vi "GetSettings.vi"(8 "error in (no error)":errorcluster, 10 "SettingsToRetrieve":variant, 11 "PacificPowerSource in":refnum<class "PacificPowerSource.lvclass">) -> (0 "error out":errorcluster, 1 "DeviceConfig&Meas":variant, 2 "RetrievedSettings":variant, 3 "PacificPowerSource Out":refnum<class "PacificPowerSource.lvclass">)   [LabVIEW 2018, in "AcPwrPlugins.lvlib" / "PacificPowerSource.lvclass"]
doc: "This VI retrieves a boolean status to see if the instrument can conduct measurements while the device is changing modes or turning off and on."
uses:
  PacificPowerSource.lvclass
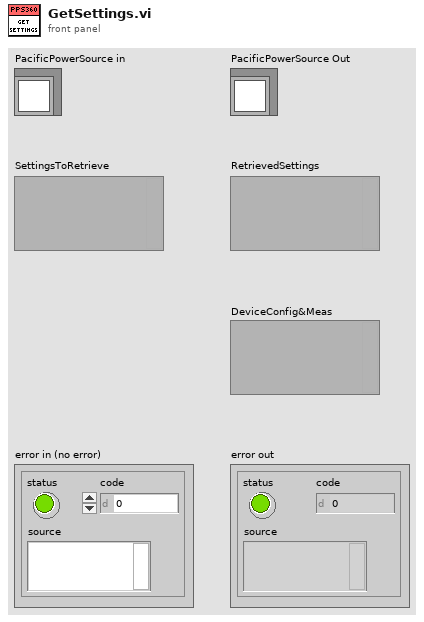
[diagram p1: front panel]
types:
  T1 = typedef "AcPwrPlugins.lvlib/PacificPowerSource.lvclass/Device(s)Settings.ctl" = cluster{"MeasName":string, "Modules":cluster{"Handle":string, "Connected":bool, "Clear Device (F)":bool, "btnIdQuery":bool, "btnReset":bool, "Program #":cluster{"Phase B (Degrees)":i32, "Waveform A (1: Sine)":i32, "Voltage Level (Va)":dbl, "Program Number (0)":i32, "Voltage Level (Vb) ":dbl, "Form (3: Three)":u16, "Coupling  (0: Direct)":u16, "Frequency (45Hz)":dbl, "Current Limit (40A)":dbl, "Phase C (Degrees)":i32, "Voltage Level (Vc)":dbl, "Waveform B (1: Sine)":i32, "Waveform C (1: Sine)":i32}[], "Impedance Parameters (off, 0.00)":cluster{"State":bool, "Impedance":dbl}, "Transient Execution (F)":bool, "OutputEnabled":bool, "Source Range":cluster{"Frequency Minimum (45 Hz)":dbl, "Frequency Maximum (1200 Hz)":dbl, "Voltage Maximum (V)":dbl, "Voltage Minimum (V)":dbl, "Range Control (0: Auto)":u16, "Initial Voltage (0V)":dbl, "Frequency Range (600Hz)":u16}, "Port Type":enum16{"GPIB", "Serial"}}[]}
  T2 = typedef "AcPwrPlugins.lvlib/PacificPowerSource.lvclass/Measurements.ctl" = cluster{"Handle":string, "Name":string, "Enabled ":bool, "Measurement Value":dbl, "Channel Name":enum16{"A", "B", "C"}, "Measurement Type ":T3}[]
  T3 = typedef "AcPwrPlugins.lvlib/PacificPowerSource.lvclass/MeasurementType.ctl" = enum16{"Voltage RMS L-N", "Voltage RMS L-L", "Frequency", "Current RMS", "Current Peak", "Crest Factor", "Power Factor", "Power VA", "Real Power"}
  T4 = cluster{"xml string":string, "xml string":string}
  T5 = cluster{"Device(s)Settings":T1, "Measurements":T2}
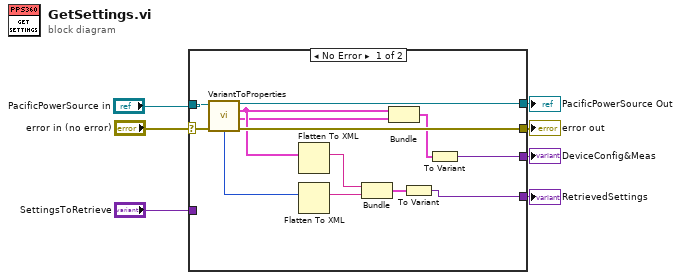
[diagram p0: block diagram]
diagram:
  n1 = case shown="No Error" "error in (no error)" {
    selector: "error in (no error)" -> [w19 w22]
    tunnel: "PacificPowerSource in" -> [w20 w23]
    tunnel: [w18 w23] -> w4
    tunnel: [w17 w22] -> w3
    tunnel: "SettingsToRetrieve" -> [_ w21]
    tunnel: [w12 w21] -> w2
    tunnel: [w8 _] -> w1
    frame No Error {
      n2 = call "VariantToProperties.vi"("PacificPowerSource in"=w20, "error in (no error)"=w19) -> ("PacificPowerSource out"=w18:refnum<class "PacificPowerSource.lvclass">, "Device(s)Settings"=w11:T1, "Measurements"=w10:T2, "Measurement Refresh Time (ms)"=w13:u32, "error out"=w17:errorcluster)  [unwired: 7 in, 2 out]
      n3 = Flatten To XML(anything=w11) -> (xml string=w15:string)
      n4 = Flatten To XML(anything=w13) -> (xml string=w14:string)
      n5 = Bundle("xml string"=w15, "xml string"=w14) -> (w16:T4)  [unwired: 1 in]
      n6 = Bundle("Device(s)Settings"=w11, "Measurements"=w10) -> (w9:T5)  [unwired: 1 in]
      n7 = To Variant(anything=w16) -> (Variant=w12:variant)
      n8 = To Variant(anything=w9) -> (Variant=w8:variant)
    }
    frame Error {
    }
  }
  "error out" <- w3
  "PacificPowerSource Out" <- w4
  "RetrievedSettings" <- w2
  "DeviceConfig&Meas" <- w1
